vi "Find.vi"(2 "Key":string, 3 "Key-Value Pairs":cluster{"Key":string, "Value":string}[](array[cluster])) -> (0 "Found?":bool, 1 "Value":string)   [LabVIEW 2018, in "Toolkit.lvlib" / "Loaders.lvlib" / "String.lvclass"]
uses:
  String.lvclass
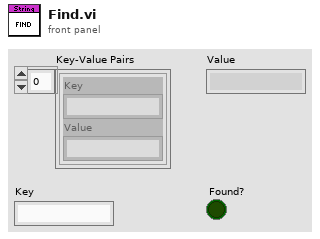
[diagram p1: front panel]
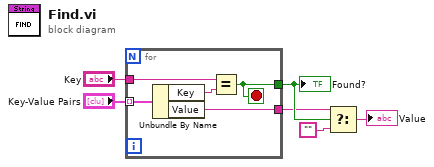
[diagram p0: block diagram]
diagram:
  n1 = for {
    tunnel: "Key-Value Pairs" -> [w11] mode=indexing
    tunnel: "Key" -> [w10]
    tunnel: [w8] -> w2
    tunnel: [w7] -> w5
    stop <- w7 stop-if-true
    n2 = Unbundle By Name(w11) -> ("Key"=w9:string, "Value"=w8:string)
    n3 = Equal?(x=w10, y=w9) -> (x = y?=w7:bool)
  }
  "Found?" <- w5
  n4 = Select(t=w2, s=w5, f="") -> (s? t:f=→"Value":string)
